vi "Read Input & Reset.vi"(8 "error in (no error)":errorcluster, 11 "CAP1208 in":refnum<class "CAP1208.lvclass">) -> (0 "error out":errorcluster, 1 "Sensor Input (U8)":u8, 2 "Sensor Input (CS1-CS8)":bool[](array[boolean]), 3 "CAP1208 out":refnum<class "CAP1208.lvclass">)   [LabVIEW 2020, in "CAP1208.lvclass"]
doc: "Reads the sensor input status register and resets the interrupt flag. The chip latches button touches."
uses:
  CAP1208.lvclass
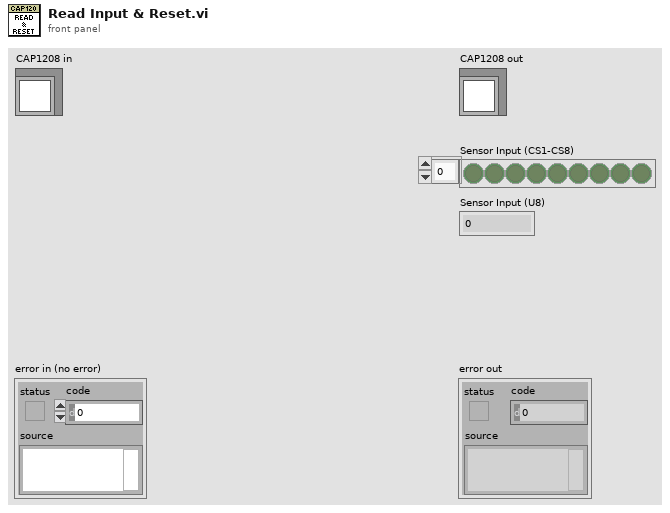
[diagram p1: front panel]
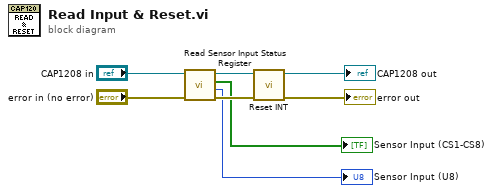
[diagram p0: block diagram]
diagram:
  n1 = call "Read Sensor Input Status Register.vi"("error in (no error)"="error in (no error)", "CAP1208 in"="CAP1208 in") -> ("error out"=w7:errorcluster, "Sensor Input (U8)"=→"Sensor Input (U8)":u8, "Sensor Input (CS1-CS8)"=→"Sensor Input (CS1-CS8)":bool[], "CAP1208 out"=w6:refnum<class "CAP1208.lvclass">)  [unwired: 6 in]
  n2 = call "Reset INT.vi"("error in (no error)"=w7, "CAP1208 in"=w6) -> ("error out"=→"error out":errorcluster, "CAP1208 out"=→"CAP1208 out":refnum<class "CAP1208.lvclass">)  [unwired: 8 in]
